vi "CloseEQE_ActiveX.vi"(6 "Skip?":bool, 8 "error in (no error)":errorcluster) -> (0 "error out":errorcluster)   [LabVIEW 2016]
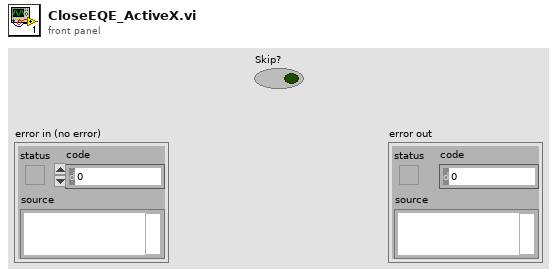
[diagram p1: front panel]
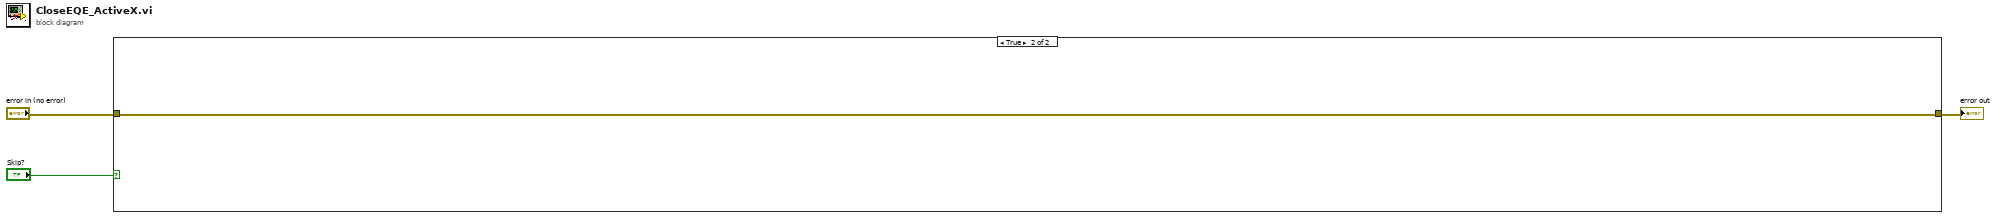
[diagram p0: block diagram]
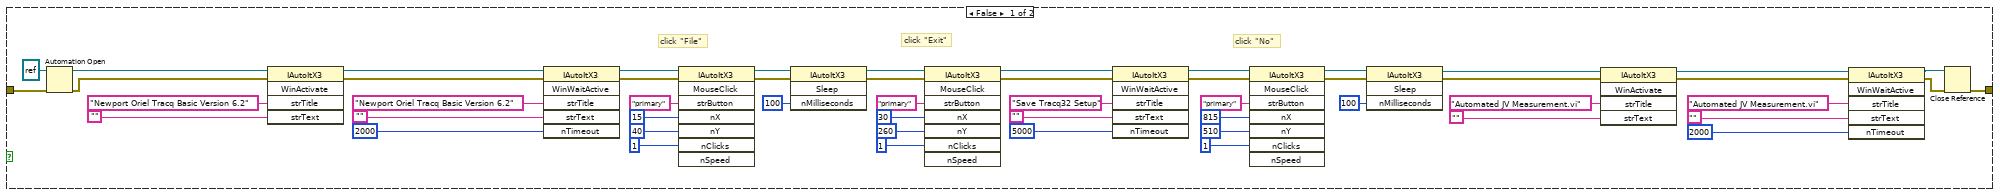
[diagram p2: hidden frame]
diagram:
  n1 = case shown="True" "Skip?" {
    tunnel: "error in (no error)" -> [w54 w56]
    tunnel: [w53 w56] -> w2
    frame False {
      # "click \"No\""
      # "click \"Exit\""
      # "click \"File\""
      n2 = Automation Open(error in (no error)=w54, Automation Refnum=refnum<k7> refnum ("AutoItX3Lib.IAutoItX3")) -> (Automation Refnum=w21:refnum<k7>, error out=w20:errorcluster)  [unwired: 2 in]
      n3 = invoke class="IAutoItX3" method="WinActivate"(reference=w21, error in=w20, "strTitle"="Newport Oriel Tracq Basic Version 6.2", "strText"="") -> (reference out=w52:refnum<k7>, error out=w45:errorcluster)  [unwired: 1 in, 3 out]
      n4 = invoke class="IAutoItX3" method="WinWaitActive"(reference=w52, error in=w45, "strTitle"="Newport Oriel Tracq Basic Version 6.2", "strText"="", "nTimeout"=2000) -> (reference out=w46:refnum<k7>, error out=w44:errorcluster)  [unwired: 1 in, 4 out]
      n5 = invoke class="IAutoItX3" method="MouseClick"(reference=w46, error in=w44, "strButton"="primary", "nX"=15, "nY"=40, "nClicks"=1) -> (reference out=w38:refnum<k7>, error out=w37:errorcluster)  [unwired: 2 in, 6 out]
      n6 = invoke class="IAutoItX3" method="Sleep"(reference=w38, error in=w37, "nMilliseconds"=100) -> (reference out=w32:refnum<k7>, error out=w31:errorcluster)  [unwired: 1 in, 2 out]
      n7 = invoke class="IAutoItX3" method="MouseClick"(reference=w32, error in=w31, "strButton"="primary", "nX"=30, "nY"=260, "nClicks"=1) -> (reference out=w27:refnum<k7>, error out=w26:errorcluster)  [unwired: 2 in, 6 out]
      n8 = invoke class="IAutoItX3" method="WinWaitActive"(reference=w27, error in=w26, "strTitle"="Save Tracq32 Setup", "strText"="", "nTimeout"=5000) -> (reference out=w19:refnum<k7>, error out=w18:errorcluster)  [unwired: 1 in, 4 out]
      n9 = invoke class="IAutoItX3" method="MouseClick"(reference=w19, error in=w18, "strButton"="primary", "nX"=815, "nY"=510, "nClicks"=1) -> (reference out=w16:refnum<k7>, error out=w15:errorcluster)  [unwired: 2 in, 6 out]
      n10 = invoke class="IAutoItX3" method="Sleep"(reference=w16, error in=w15, "nMilliseconds"=100) -> (reference out=w7:refnum<k7>, error out=w6:errorcluster)  [unwired: 1 in, 2 out]
      n11 = invoke class="IAutoItX3" method="WinActivate"(reference=w7, error in=w6, "strTitle"="Automated JV Measurement.vi", "strText"="") -> (reference out=w14:refnum<k7>, error out=w8:errorcluster)  [unwired: 1 in, 3 out]
      n12 = invoke class="IAutoItX3" method="WinWaitActive"(reference=w14, error in=w8, "strTitle"="Automated JV Measurement.vi", "strText"="", "nTimeout"=2000) -> (reference out=w5:refnum<k7>, error out=w4:errorcluster)  [unwired: 1 in, 4 out]
      n13 = Close Reference(reference=w5, error in (no error)=w4) -> (error out=w53:errorcluster)
    }
    frame True {
    }
  }
  "error out" <- w2
